vi "Finish.vi"   [LabVIEW 2016]
doc: "This VI is called just before exiting. It is expected to close I/O refnum, save collected data, etc."
uses:
  <vilib>/Rock Robotics/WPI/Utilities/WPI_GetSetVariantRefNum.vi
  navX Library v2/navX Library v2.lvlib
types:
  T1 = typedef "WPI_PotentiometerDevRef.ctl" = cluster{"DevStatus":errorcluster, "Analog Channel":T2, "Invert Output":bool}
  T2 = typedef "FPGA_AIChannel.ctl" = enum8{"AI 0", "AI 1", "AI 2", "AI 3", "AI MXP 0", "AI MXP 1", "AI MXP 2", "AI MXP 3", "Invalid"}
  T3 = typedef "WPI_MotorControlDeviceRef.ctl" = cluster{"DeviceStatus":errorcluster, "Type":T4, "PWM":cluster{"PWM Channel":T5, "DeadBand":T6}, "CAN":cluster{"Device Number":u8, "SetOutput VI Ref":variant, "GetOutput VI Ref":variant, "Enable VI Ref":variant, "Disable VI Ref":variant, "Data":variant}, "Invert":bool}
  T4 = typedef "WPI_MotorControlType.ctl" = enum16{"PWM", "CAN"}
  T5 = typedef "FPGA_DIOPWMChannel.ctl" = enum8{"PWM 0", "PWM 1", "PWM 2", "PWM 3", "PWM 4", "PWM 5", "PWM 6", "PWM 7", "PWM 8", "PWM 9", "PWM MXP 0", "PWM MXP 1", "PWM MXP 2", "PWM MXP 3", "PWM MXP 4", "PWM MXP 5", "PWM MXP 6", "PWM MXP 7", "PWM MXP 8", "PWM MXP 9", "Invalid"}
  T6 = typedef "WPI_PWMDeadband.ctl" = cluster{"Name":string, "maxPositivePwm":i32, "minPositivePwm":i32, "centerPwm":i32, "maxNegativePwm":i32, "minNegativePwm":i32, "angularRange":u16}
  T7 = typedef "WPI_EncoderDevRef.ctl" = cluster{"DevStatus":errorcluster, "EncoderIndex":T8, "CounterIndex":T9, "DistancePerCount":dbl, "Decoding Type":T10}
  T8 = typedef "FPGA_EncoderIdx.ctl" = enum8{"Enc 0", "Enc 1", "Enc 2", "Enc 3", "Enc 4", "Enc 5", "Enc 6", "Enc 7", "Invalid"}
  T9 = typedef "FPGA_CounterCtrSystemIndex.ctl" = enum8{"Ctr 0", "Ctr 1", "Ctr 2", "Ctr 3", "Ctr 4", "Ctr 5", "Ctr 6", "Ctr 7", "Invalid"}
  T10 = typedef "WPI_EncoderType.ctl" = enum16{"1x", "2x", "4x"}
  T11 = typedef "WPI_JoystickDevRef.ctl" = cluster{"Device":T12}
  T12 = typedef "WPI_JoystickDeviceEnum.ctl" = enum16{"USB 0", "USB 1", "USB 2", "USB 3", "USB 4", "USB 5"}
  T13 = typedef "WPI_RobotDriveDevRef.ctl" = cluster{"DevStatus":errorcluster, "Motors[]":T3[], "Square Inputs":bool, "Max Output":dbl}
  T14 = typedef "navX Library v2.lvlib/Z900_navX_DeviceTypeDef.ctl" = cluster{"Interface":cluster{"Protocol":T15, "Update Rate (4Hz-100Hz)":u8, "navX Open TypeDef":variant}, "Notify Packet":refnum<notifier>, "Loop VI Refnum":refnum<vi>, "Ready to Close Occurrence Refnum":refnum<k4>}
  T15 = typedef "navX Library v2.lvlib/Z900_navX_ProtocolTypeDef.ctl" = enum16{"SERIAL", "I2C", "SPI"}
  T16 = typedef "WPI_CompressorDevRef.ctl" = cluster{"DevStatus":errorcluster, "Pneumatics Control Module":u8}
  T17 = typedef "WPI_SolenoidDevRef.ctl" = cluster{"DevStatus":errorcluster, "Pneumatics Control Module":u8, "Forward Solenoid Channel":T18, "Reverse Solenoid Channel":T18}
  T18 = typedef "WPI_SolenoidChannel.ctl" = enum8{"Solenoid 0", "Solenoid 1", "Solenoid 2", "Solenoid 3", "Solenoid 4", "Solenoid 5", "Solenoid 6", "Solenoid 7", "Invalid"}
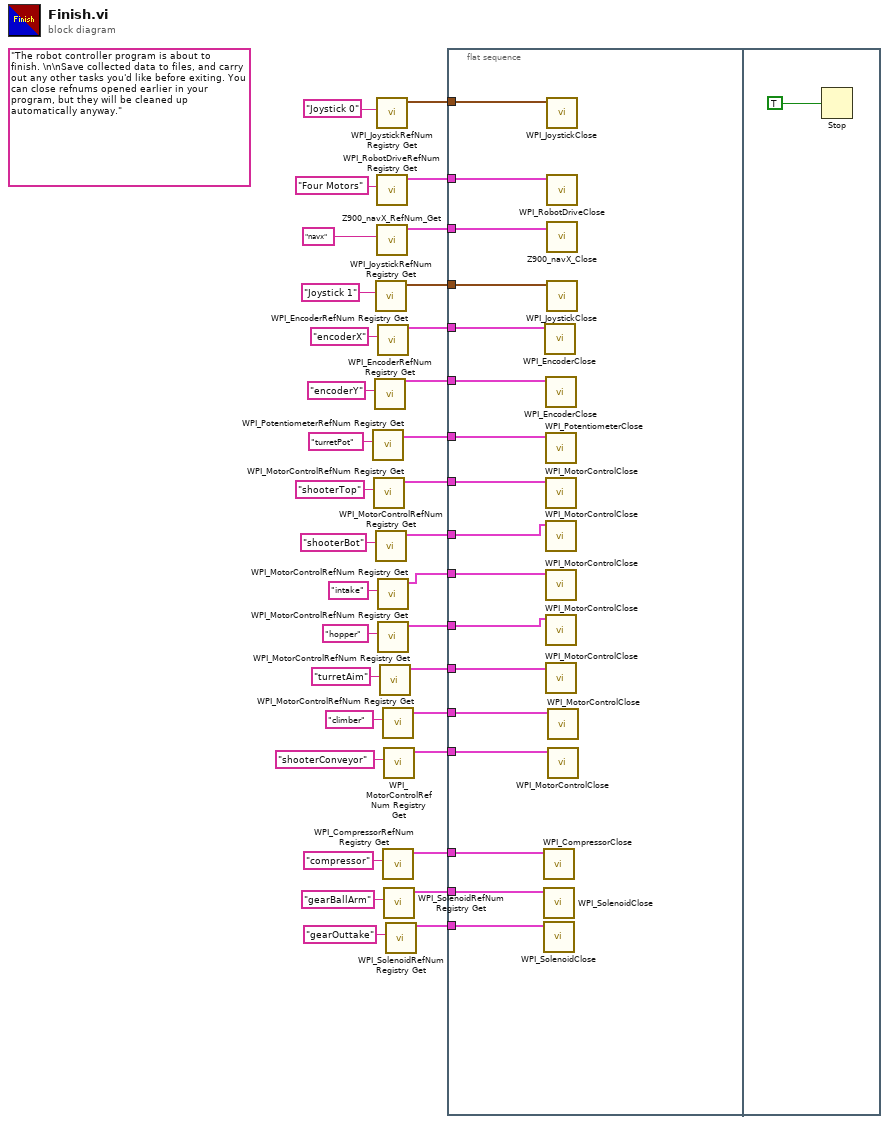
[diagram p0: block diagram]
diagram:
  (unwired) "The robot controller program is about to finish. \n\nSave collected data to files, and carry out any other tasks you'd like before exiting. You can close refnums opened earlier in your program, but they will be cleaned up automatically anyway."
  n1 = call <vilib>:"WPI_PotentiometerRefNum Registry Get.vi"("refnum name"="turretPot") -> ("PotDevRef"=w22:T1)  [unwired: 9 in, 1 out]
  n2 = call <vilib>:"WPI_MotorControlRefNum Registry Get.vi"("refnum name"="shooterTop") -> ("MotorControlDevRef"=w20:T3)  [unwired: 9 in, 1 out]
  n3 = call <vilib>:"WPI_EncoderRefNum Registry Get.vi"("refnum name"="encoderY") -> ("EncoderDevRef"=w24:T7)  [unwired: 9 in, 1 out]
  n4 = call <vilib>:"WPI_JoystickRefNum Registry Get.vi"("refnum name"="Joystick 1") -> ("JoystickDevRef"=w27:T11)  [unwired: 1 in, 9 out]
  n5 = call <vilib>:"WPI_MotorControlRefNum Registry Get.vi"("refnum name"="shooterBot") -> ("MotorControlDevRef"=w13:T3)  [unwired: 9 in, 1 out]
  n6 = call <vilib>:"WPI_JoystickRefNum Registry Get.vi"("refnum name"="Joystick 0") -> ("JoystickDevRef"=w31:T11)  [unwired: 1 in, 9 out]
  n7 = call <vilib>:"WPI_RobotDriveRefNum Registry Get.vi"("refnum name"="Four Motors") -> ("RobotDriveDevRef"=w32:T13)  [unwired: 1 in, 9 out]
  n8 = call "Z900_navX_RefNum_Get.vi"("refnum name"="navx") -> ("navX Device"=w30:T14)  [unwired: 9 in, 1 out]
  n9 = call <vilib>:"WPI_EncoderRefNum Registry Get.vi"("refnum name"="encoderX") -> ("EncoderDevRef"=w25:T7)  [unwired: 9 in, 1 out]
  n10 = call <vilib>:"WPI_MotorControlRefNum Registry Get.vi"("refnum name"="intake") -> ("MotorControlDevRef"=w12:T3)  [unwired: 9 in, 1 out]
  n11 = call <vilib>:"WPI_MotorControlRefNum Registry Get.vi"("refnum name"="hopper") -> ("MotorControlDevRef"=w11:T3)  [unwired: 9 in, 1 out]
  n12 = call <vilib>:"WPI_MotorControlRefNum Registry Get.vi"("refnum name"="turretAim") -> ("MotorControlDevRef"=w10:T3)  [unwired: 9 in, 1 out]
  n13 = call <vilib>:"WPI_MotorControlRefNum Registry Get.vi"("refnum name"="climber") -> ("MotorControlDevRef"=w9:T3)  [unwired: 9 in, 1 out]
  n14 = call <vilib>:"WPI_CompressorRefNum Registry Get.vi"("refnum name"="compressor") -> ("CompressorDevRef"=w6:T16)  [unwired: 9 in, 1 out]
  n15 = call <vilib>:"WPI_MotorControlRefNum Registry Get.vi"("refnum name"="shooterConveyor") -> ("MotorControlDevRef"=w7:T3)  [unwired: 9 in, 1 out]
  n16 = call <vilib>:"WPI_SolenoidRefNum Registry Get.vi"("refnum name"="gearBallArm") -> ("SolenoidDevRef"=w4:T17)  [unwired: 9 in, 1 out]
  n17 = call <vilib>:"WPI_SolenoidRefNum Registry Get.vi"("refnum name"="gearOuttake") -> ("SolenoidDevRef"=w1:T17)  [unwired: 9 in, 1 out]
  n18 = flat-sequence {
    tunnel: w32 -> [w51]
    tunnel: w31 -> [w50]
    tunnel: w30 -> [w49]
    tunnel: w27 -> [w48]
    tunnel: w25 -> [w47]
    tunnel: w24 -> [w46]
    tunnel: w22 -> [w45]
    tunnel: w20 -> [w44]
    tunnel: w13 -> [w43]
    tunnel: w12 -> [w42]
    tunnel: w11 -> [w41]
    tunnel: w10 -> [w40]
    tunnel: w9 -> [w39]
    tunnel: w7 -> [w38]
    tunnel: w6 -> [w37]
    tunnel: w4 -> [w36]
    tunnel: w1 -> [w35]
    frame #0 {
      n19 = call <vilib>:"WPI_CompressorClose.vi"("CompressorDevRef"=w37) -> ()  [unwired: 10 in, 1 out]
      n20 = call <vilib>:"WPI_SolenoidClose.vi"("SolenoidDevRef"=w36) -> ()  [unwired: 10 in, 1 out]
      n21 = call <vilib>:"WPI_SolenoidClose.vi"("SolenoidDevRef"=w35) -> ()  [unwired: 10 in, 1 out]
      n22 = call <vilib>:"WPI_EncoderClose.vi"("EncoderDevRef"=w47) -> ()  [unwired: 10 in, 1 out]
      n23 = call <vilib>:"WPI_EncoderClose.vi"("EncoderDevRef"=w46) -> ()  [unwired: 10 in, 1 out]
      n24 = call <vilib>:"WPI_PotentiometerClose.vi"("PotDevRef"=w45) -> ()  [unwired: 10 in, 1 out]
      n25 = call <vilib>:"WPI_MotorControlClose.vi"("MotorControlDevRef"=w44) -> ()  [unwired: 10 in, 1 out]
      n26 = call <vilib>:"WPI_MotorControlClose.vi"("MotorControlDevRef"=w43) -> ()  [unwired: 10 in, 1 out]
      n27 = call <vilib>:"WPI_MotorControlClose.vi"("MotorControlDevRef"=w42) -> ()  [unwired: 10 in, 1 out]
      n28 = call <vilib>:"WPI_MotorControlClose.vi"("MotorControlDevRef"=w41) -> ()  [unwired: 10 in, 1 out]
      n29 = call <vilib>:"WPI_MotorControlClose.vi"("MotorControlDevRef"=w40) -> ()  [unwired: 10 in, 1 out]
      n30 = call <vilib>:"WPI_JoystickClose.vi"("JoystickDevRef"=w50) -> ()  [unwired: 11 out]
      n31 = call <vilib>:"WPI_RobotDriveClose.vi"("RobotDriveDevRef"=w51) -> ()  [unwired: 1 in, 10 out]
      n32 = call "Z900_navX_Close.vi"("navX Device"=w49) -> ()  [unwired: 10 in, 1 out]
      n33 = call <vilib>:"WPI_JoystickClose.vi"("JoystickDevRef"=w48) -> ()  [unwired: 11 out]
      n34 = call <vilib>:"WPI_MotorControlClose.vi"("MotorControlDevRef"=w39) -> ()  [unwired: 10 in, 1 out]
      n35 = call <vilib>:"WPI_MotorControlClose.vi"("MotorControlDevRef"=w38) -> ()  [unwired: 10 in, 1 out]
    }
    frame #1 {
      n36 = Stop(stop? (T)=TRUE ("Quit")) -> ()
    }
  }
